vi "Read UserEventDLCommand.vi"(8 "error in (no error)":errorcluster caption="entrée d'erreur (pas d'erreur)", 11 "DelayLine en entrée":refnum<class "DelayLine.lvclass">) -> (0 "error out":errorcluster caption="sortie d'erreur", 2 "UserEventDLCommand":refnum<user-event>, 3 "DelayLine en sortie":refnum<class "DelayLine.lvclass">)   [LabVIEW 2015]
uses:
  DelayLine.lvclass
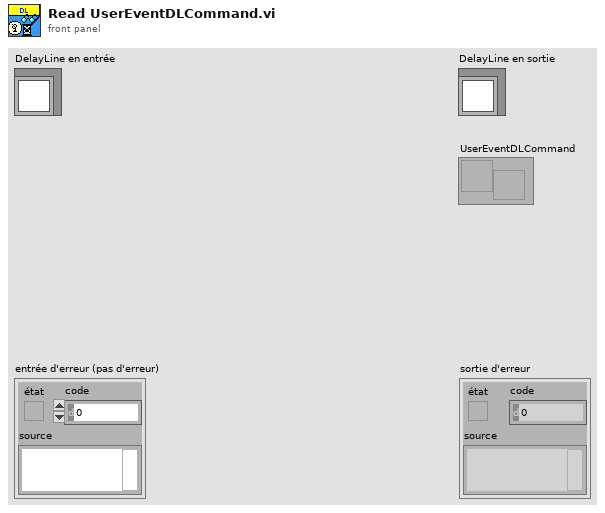
[diagram p1: front panel]
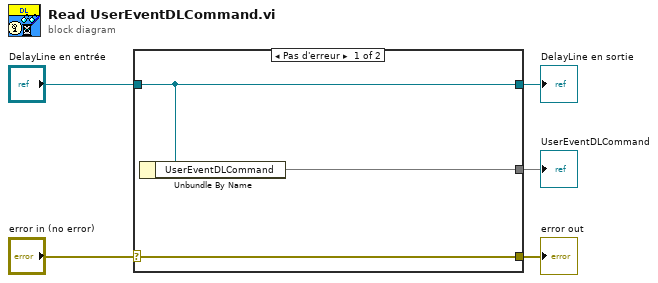
[diagram p0: block diagram]
diagram:
  n1 = case shown="Pas d'erreur" "error in (no error)" {
    selector: "error in (no error)" -> [w8 w9]
    tunnel: [w8 w9] -> w4
    tunnel: [w7 w10] -> w2
    tunnel: "DelayLine en entrée" -> [w7 w10]
    tunnel: [w6 _] -> w1
    frame No Error {
      n2 = Unbundle By Name(w7) -> ("UserEventDLCommand"=w6)
    }
    frame Error {
    }
  }
  "error out" <- w4
  "DelayLine en sortie" <- w2
  "UserEventDLCommand" <- w1
